vi "UIRef.vi"(8 "error in":errorcluster, 11 "Getting Started IO editor node in":refnum<class "io editor node.lvclass">) -> (0 "error out":errorcluster, 2 "VI refnum":refnum<vi>, 3 "Getting Started IO editor node out":refnum<class "io editor node.lvclass">)   [LabVIEW 2014, in "io editor node.lvclass"]
uses:
  io editor node.lvclass
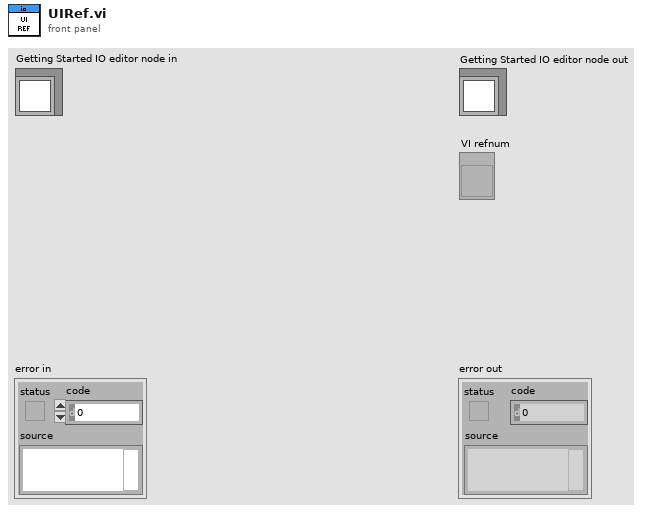
[diagram p1: front panel]
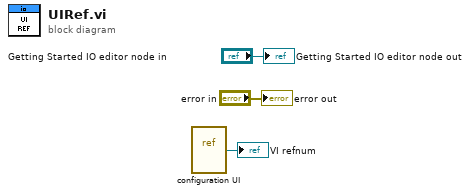
[diagram p0: block diagram]
diagram:
  n1 = vi-ref "configuration UI.vi"() -> (→"VI refnum":refnum<vi>)
  "error out" <- "error in"
  "Getting Started IO editor node out" <- "Getting Started IO editor node in"
